vi "调整窗口大小.vi"(0 "前面板窗口:前面板边界":T1, 1 "x":i16=1024, 2 "y":i16=591) -> (7 "前面板边界":T1)   [LabVIEW 2018]
uses:
  <vilib>/Utility/miscctls.llb/LVRectTypeDef.ctl
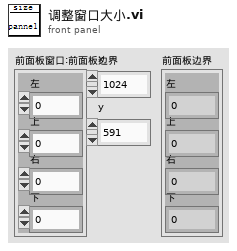
[diagram p1: front panel]
types:
  T1 = typedef "LVRectTypeDef.ctl" = cluster{"Left":i16, "Top":i16, "Right":i16, "Bottom":i16}
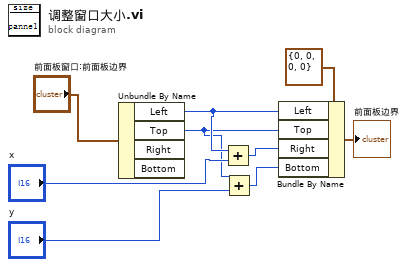
[diagram p0: block diagram]
diagram:
  n1 = Unbundle By Name("前面板窗口:前面板边界") -> ("Left"=w9:i16, "Top"=w5:i16)  [unwired: 2 out]
  n2 = Add(x=w9, y="x") -> (x+y=w7:i16)
  n3 = Add(x=w5, y="y") -> (x+y=w6:i16)
  n4 = Bundle By Name(cluster=T1 {"Left"=0, "Top"=0, "Right"=0, "Bottom"=0} ("前面板窗口:前面板边界"), "Left"=w9, "Top"=w5, "Right"=w7, "Bottom"=w6) -> (→"前面板边界":T1)
